vi "Obtain Control Cluster.vi"(9 "I/O":bool=TRUE, 10 "Dispense":bool=TRUE, 11 "Motion":bool=TRUE) -> (3 "Control Out":T1)   [LabVIEW 2016, in "Controller.lvclass"]
uses:
  Controller.lvclass
  Controllers.ctl
  I-O/I-O.lvclass
  Motion/A3200/A3200.lvclass
  C:/Users/HEP Gantry/Documents/Assembly/Assembly Folder/V4/Classes/Controller/Motion/Motion.lvclass
  Dispenser/Dispenser.lvclass
  Motion/Motion.lvclass
  Dispenser/Ultimus V/Ultimus V.lvclass
  C:/Users/HEP Gantry/Documents/Assembly/Assembly Folder/V4/Classes/Controller/Dispenser/Dispenser.lvclass
  I-O/NI-DAQ/NI-DAQ.lvclass
  C:/Users/HEP Gantry/Documents/Assembly/Assembly Folder/V4/Classes/Controller/I-O/I-O.lvclass
panel:
  in  "Control":T1={"I-O.lvclass"=refnum, "Motion.lvclass"=refnum, "Dispenser.lvclass"=refnum}
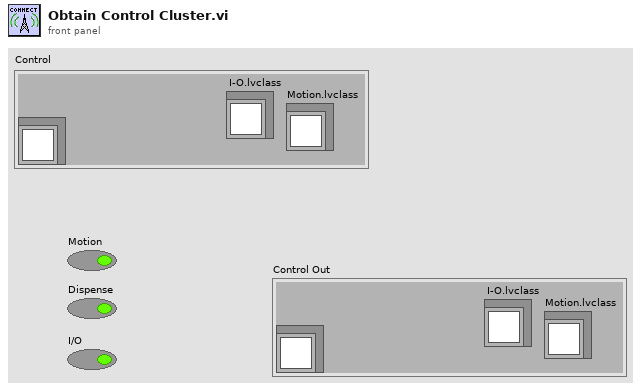
[diagram p1: front panel]
types:
  T1 = typedef "Controller.lvclass/Controllers.ctl" = cluster{"I-O.lvclass":refnum<class "I-O.lvclass">, "Motion.lvclass":refnum<class "Motion.lvclass">, "Dispenser.lvclass":refnum<class "Dispenser.lvclass">}
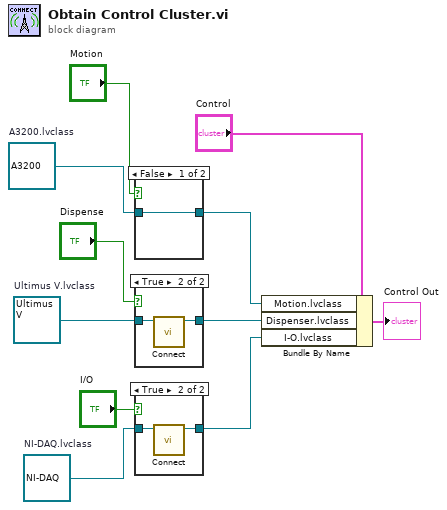
[diagram p0: block diagram]
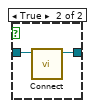
[diagram p2: hidden frame]
diagram:
  w1 = refnum<class "NI-DAQ.lvclass"> refnum  # NI-DAQ.lvclass
  w8 = refnum<class "A3200.lvclass"> refnum  # A3200.lvclass
  w9 = refnum<class "Ultimus V.lvclass"> refnum  # Ultimus V.lvclass
  n1 = case shown="False" "Motion" {
    tunnel: [w12 w14] -> w11
    tunnel: w8 -> [w12 w13]
    frame False {
    }
    frame True {
      n2 = call-dynamic "Connect.vi"("Gantry in"=w13) -> ("Gantry out"=w14:refnum<class "A3200.lvclass">)  [unwired: 9 in, 1 out]
    }
  }
  n3 = case shown="True" "Dispense" {
    tunnel: [w15 w17] -> w10
    tunnel: w9 -> [w15 w16]
    frame False {
    }
    frame True {
      n4 = call-dynamic "Connect.vi"("Ultimus V in"=w16) -> ("Ultimus V out"=w17:refnum<class "Ultimus V.lvclass">)  [unwired: 9 in, 1 out]
    }
  }
  n5 = case shown="True" "I/O" {
    tunnel: w1 -> [w18 w20]
    tunnel: [w18 w19] -> w5
    frame False {
    }
    frame True {
      n6 = call-dynamic "Connect.vi"("NI-DAQ in"=w20) -> ("NI-DAQ out"=w19:refnum<class "NI-DAQ.lvclass">)  [unwired: 9 in, 1 out]
    }
  }
  n7 = Bundle By Name(cluster="Control", "Motion.lvclass"=w11, "Dispenser.lvclass"=w10, "I-O.lvclass"=w5) -> (→"Control Out":T1)
